vi "Read Motor Velocity.vi"(8 "error in (no error)":errorcluster, 10 "Motor ID (0)":u8, 11 "Dynamixel Motor VISA in":refnum<class "Dynamixel Motor VISA.lvclass">) -> (0 "error out":errorcluster, 2 "Velocity (RPM)":dbl, 3 "Dynamixel Motor VISA out":refnum<class "Dynamixel Motor VISA.lvclass">)   [LabVIEW 2016, in "Dynamixel Motor VISA.lvclass"]
doc: "Retrieves the motor's velocity."
uses:
  <instrlib>/Dynamixel Motor/HAIOL/VISA/Dynamixel Motor VISA.lvclass
  <instrlib>/Dynamixel Motor/HAIOL/VISA/Dynamixel Motor VISA.lvclass/Dynamixel Motor VISA.ctl
  <instrlib>/Dynamixel Motor/Dynamixel Motor.lvlib
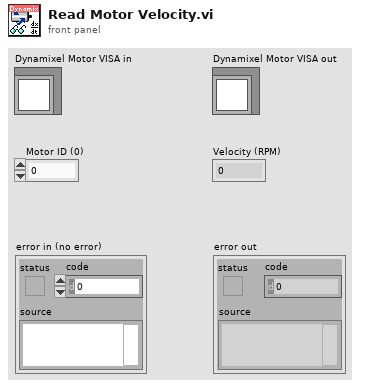
[diagram p1: front panel]
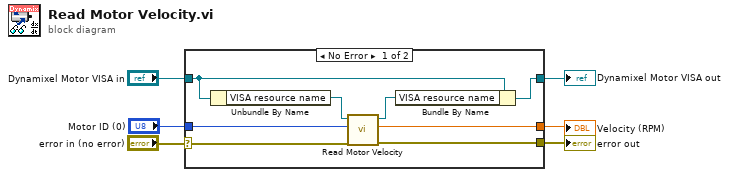
[diagram p0: block diagram]
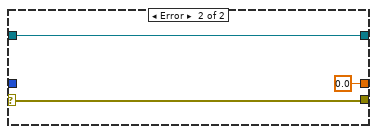
[diagram p2: hidden frame]
diagram:
  n1 = case shown="No Error" "error in (no error)" {
    selector: "error in (no error)" -> [w14 w16]
    tunnel: "Dynamixel Motor VISA in" -> [w10 w17]
    tunnel: "Motor ID (0)" -> [w13 _]
    tunnel: [w11 w16] -> w3
    tunnel: [w8 w17] -> w2
    tunnel: [w7 0.0 ("Velocity (RPM)")] -> w1
    frame No Error {
      n2 = Unbundle By Name(w10) -> ("VISA resource name"=w12:refnum<visa-resource-name>)
      n3 = call <instrlib>:"Read Motor Velocity.vi"("error in (no error)"=w14, "Motor ID (0)"=w13, "VISA resource name"=w12) -> ("error out"=w11:errorcluster, "Velocity (RPM)"=w7:dbl, "VISA resource name out"=w9:refnum<visa-resource-name>)  [unwired: 6 in]
      n4 = Bundle By Name(cluster=w10, "VISA resource name"=w9) -> (w8:refnum<class "Dynamixel Motor VISA.lvclass">)
    }
    frame Error {
    }
  }
  "error out" <- w3
  "Dynamixel Motor VISA out" <- w2
  "Velocity (RPM)" <- w1
